vi "点到线距离.vi"(9 "点坐标":cluster{"Numeric":dbl, "Numeric":dbl}, 10 "Straight Edge (Find Straight Edge 1)":T2, 11 "引用句柄输入":T3) -> (1 "Distance":dbl, 2 "垂点坐标":cluster{"X":sgl, "Y":sgl})   [LabVIEW 2014]
uses:
  <vilib>/vision/Image Controls.llb/IMAQ Image.ctl
  <vilib>/vision/NI_Vision_Development_Module.lvlib
panel:
  in  "Width":i32=25
  out "Perpendicular Line":T1
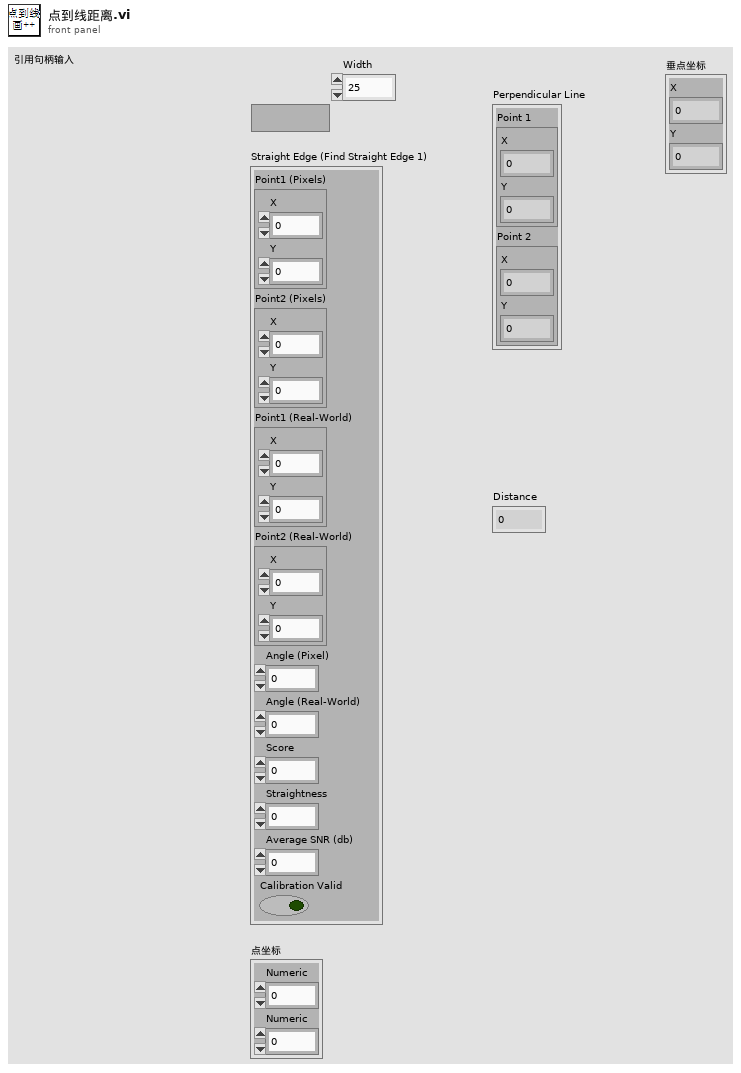
[diagram p1: front panel]
types:
  T1 = cluster{"Point 1":cluster{"X":sgl, "Y":sgl}, "Point 2":cluster{"X":sgl, "Y":sgl}}
  T2 = cluster{"Point1 (Pixels)":cluster{"X":sgl, "Y":sgl}, "Point2 (Pixels)":cluster{"X":sgl, "Y":sgl}, "Point1 (Real-World)":cluster{"X":sgl, "Y":sgl}, "Point2 (Real-World)":cluster{"X":sgl, "Y":sgl}, "Angle (Pixel)":dbl, "Angle (Real-World)":dbl, "Score":dbl, "Straightness":dbl, "Average SNR (db)":dbl, "Calibration Valid":bool}
  T3 = typedef "IMAQ Image.ctl" = refnum<image>
  T4 = cluster{"Point1 (Pixels)":cluster{"X":sgl, "Y":sgl}, "Point2 (Pixels)":cluster{"X":sgl, "Y":sgl}}
  T5 = cluster{"点坐标":cluster{"Numeric":dbl, "Numeric":dbl}, "Point 2":cluster{"X":sgl, "Y":sgl}}
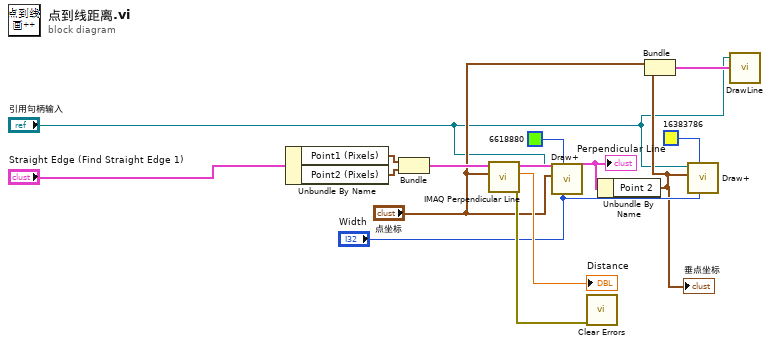
[diagram p0: block diagram]
diagram:
  n1 = Unbundle By Name("Straight Edge (Find Straight Edge 1)") -> ("Point1 (Pixels)"=w13:cluster{"X":sgl, "Y":sgl}, "Point2 (Pixels)"=w12:cluster{"X":sgl, "Y":sgl})
  n2 = Bundle("Point1 (Pixels)"=w13, "Point2 (Pixels)"=w12) -> (w11:T4)  [unwired: 1 in]
  n3 = call "IMAQ Perpendicular Line"("Point"="点坐标", "Line"=w11) -> ("error out"=w7:errorcluster, "Distance"=→"Distance":dbl, "Perpendicular Line"=w5:T1)  [unwired: 7 in]
  "Perpendicular Line" <- w5
  n4 = call "Draw+.vi"("Width"="Width", "Color"=u32 6618880, "input cluster"="点坐标", "Image In"="引用句柄输入") -> ()  [unwired: 2 in, 1 out]
  n5 = call <vilib>:"Clear Errors.vi"("error in (no error)"=w7) -> ()  [unwired: 5 in, 2 out]
  n6 = Unbundle By Name(w5) -> ("Point 2"=w3:cluster{"X":sgl, "Y":sgl})
  "垂点坐标" <- w3
  n7 = Bundle("点坐标"="点坐标", "Point 2"=w3) -> (w4:T5)  [unwired: 1 in]
  n8 = call "Draw+.vi"("Width"="Width", "Color"=u32 16383786, "input cluster"=w3, "Image In"="引用句柄输入") -> ()  [unwired: 2 in, 1 out]
  n9 = call "DrawLine.vi"("Edge Points"=w4, "img in"="引用句柄输入") -> ()  [unwired: 1 in, 1 out]
